vi "Ausgabefelder einfaerben.vi"(6 "Aktionen":T1, 11 "Angehängtes Array":refnum<vi>[](array[refnum])) -> ()   [LabVIEW 2020, in "allgemeine Sub-VIs.lvlib"]
uses:
  allgemeine Sub-VIs.lvlib
  Ausgabefelder einfaerben Aktionen.ctl
  Seiten/Anlagengrenzwerte/FGV Anlagengrenzwerte Aktionen.ctl
  Funktionstasten/Funktionstasten-Aktion.ctl
  Funktionstasten/Zustaende.ctl
  Seiten/Anlagengrenzwerte/Anlagengrenzwerte.lvlib
  Funktionstasten/Funktionstasten.lvlib
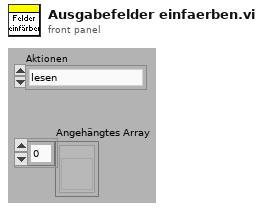
[diagram p1: front panel]
types:
  T1 = typedef "allgemeine Sub-VIs.lvlib/Ausgabefelder einfaerben Aktionen.ctl" = enum16{"lesen", "prüfen", "initialisieren"}
  T2 = typedef "Funktionstasten.lvlib/Zustaende.ctl" = enum16{"Standby", "Pause", "Eco", "Messen", "Kalibrieren", "Spülen Filter", "Spülen Leitung", "Umgebungsluft", "0-Gas", "Cal-Gas", "CG zu PNS", "-------------", "Init 1", "Init 2", "Init 3", "Init 4", "Messen vorbereiten", "Messen durchführen", "Exit"}
  T3 = typedef "Funktionstasten.lvlib/Funktionstasten-Aktion.ctl" = enum16{"Initialisieren", "Zustand setzen", "Taste gedrückt", "Fehler speichern", "Lesen", "Manuell", "Remote", "Bitparallel", "Samplepoint", "Zeit Prüfen", "reset Umschalten"}
  T4 = typedef "Anlagengrenzwerte.lvlib/FGV Anlagengrenzwerte Aktionen.ctl" = enum16{"Lesen", "Grenzwerte schreiben"}
  T5 = typedef "Anlagengrenzwerte.lvlib/Anlagen-Grenzwerte Anzeige.ctl" = cluster{"Eingangsdruck FT-IR:":T6, "Durchfluss FT-IR:":T6, "Durchfluss CalGas:":T6, "Druck Ausgang:":T6, "Druck Kalter Block:":T6, "Heizleitungen intern:":T6, "Heizleitung zu FT-IR:":T6, "Heizung Filterblock:":T6, "Heizung Pumpe:":T6, "Heizleitung Extern SP1:":T6, "Heizleitung Extern SP2:":T6, "FT-IR Heizung Messzelle:":T6, "Schaltschranktemperatur:":T6, "Gaskühler:":T6}
  T6 = typedef "Anlagengrenzwerte.lvlib/Anlagen-Parameter Anzeige.ctl" = cluster{"Sollwert":sgl, "Warn-Min":sgl, "Warn-Max":sgl, "Abschalt-Min":sgl, "Abschalt-Max":sgl, "Regler":u16}
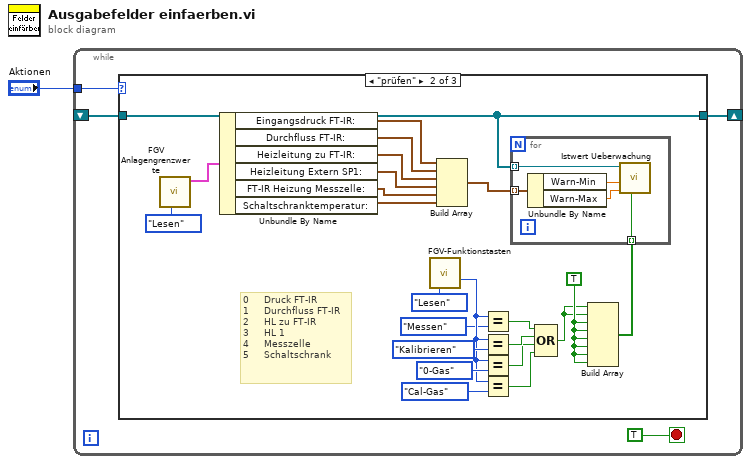
[diagram p0: block diagram]
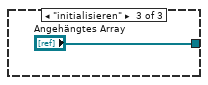
[diagram p3: hidden frame]
diagram:
  n1 = while {
    tunnel: "Aktionen" -> [w5]
    shift-right: [w4] -> _
    shift-left: _ -> [w3]
    stop <- TRUE stop-if-true
    n2 = case shown="\"prüfen\"" w5 {
      tunnel: [w6 w23 "Angehängtes Array"] -> w4
      tunnel: w3 -> [w6 w23 _]
      frame "lesen", Default {
      }
      frame "prüfen" {
        w10 = TRUE
        # "0     Druck FT-IR\n1     Durchfluss FT-IR\n2     HL zu FT-IR\n3     HL 1\n4     Messzelle\n5     Schaltschrank"
        n3 = call "FGV Anlagengrenzwerte.vi"("Aktion"=FGV_Anlagengrenzwerte_Aktionen."Lesen") -> ("Anlagen-Grenzwerte Anzeige"=w22:T5)  [unwired: 10 in]
        n4 = Unbundle By Name(w22) -> ("Eingangsdruck FT-IR:"=w29:T6, "Durchfluss FT-IR:"=w28:T6, "Heizleitung zu FT-IR:"=w27:T6, "Heizleitung Extern SP1:"=w7:T6, "FT-IR Heizung Messzelle:"=w26:T6, "Schaltschranktemperatur:"=w25:T6)
        n5 = call "FGV-Funktionstasten.vi"("Aktion"=Funktionstasten-Aktion."Lesen") -> ("ausgewählte Funktion"=w14:T2)  [unwired: 7 in, 7 out]
        n6 = Build Array(w29, w28, w27, w7, w26, w25) -> (w24:T6[])
        n7 = Equal?(x=w14, y=Zustaende."Messen") -> (x = y?=w12:bool)
        n8 = Equal?(x=w14, y=Zustaende."Kalibrieren") -> (x = y?=w20:bool)
        n9 = Equal?(x=w14, y=Zustaende."0-Gas") -> (x = y?=w19:bool)
        n10 = Equal?(x=w14, y=Zustaende."Cal-Gas") -> (x = y?=w18:bool)
        n11 = Compound Arithmetic op=OR(w12, w20, w19, w18) -> (w9:bool)
        n12 = Build Array(w9, w9, w10, w10, w10, w10, w10, w10) -> (w8:bool[])
        n13 = for {
          tunnel: w23 -> [w31] mode=indexing
          tunnel: w24 -> [w34] mode=indexing
          tunnel: w8 -> [w30] mode=indexing
          n14 = Unbundle By Name(w34) -> ("Warn-Min"=w33:sgl, "Warn-Max"=w32:sgl)
          n15 = call "Istwert Ueberwachung.vi"("Fehler Aktiviert?"=w30, "Max"=w32, "Min"=w33, "Referernz"=w31) -> ()  [unwired: 8 in]
        }
      }
      frame "initialisieren" {
      }
    }
  }
